vi "Sort Modules.vi"(8 "error in (no error)":errorcluster, 10 "Modules":refnum<class "Module.lvclass">[](array[class]), 11 "Block Diagram in":refnum<class "Block Diagram.lvclass">) -> (0 "error out":errorcluster, 3 "Block Diagram out":refnum<class "Block Diagram.lvclass">)   [LabVIEW 2015, in "Block Diagram.lvclass"]
uses:
  Block Diagram.lvclass
  Module/Module/Module.lvclass
  Block Diagram.lvclass/Block Diagram.ctl
  Structures/Structures.lvclass/Structures.ctl
  Structures/Read Name.vi
  Module Loop/Write Modules.vi
  Module Loop/Module Loop.lvclass
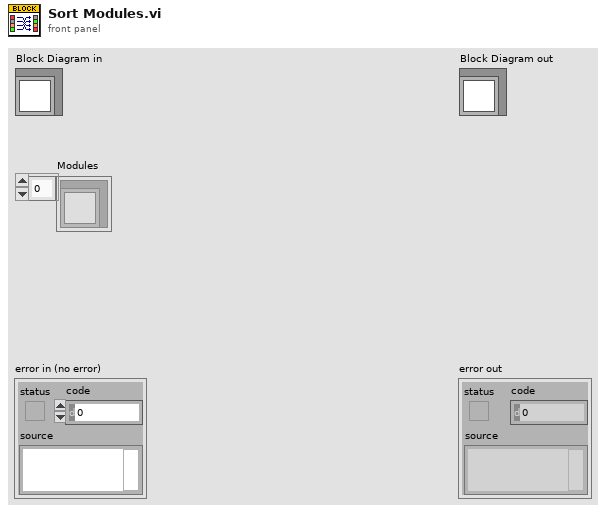
[diagram p1: front panel]
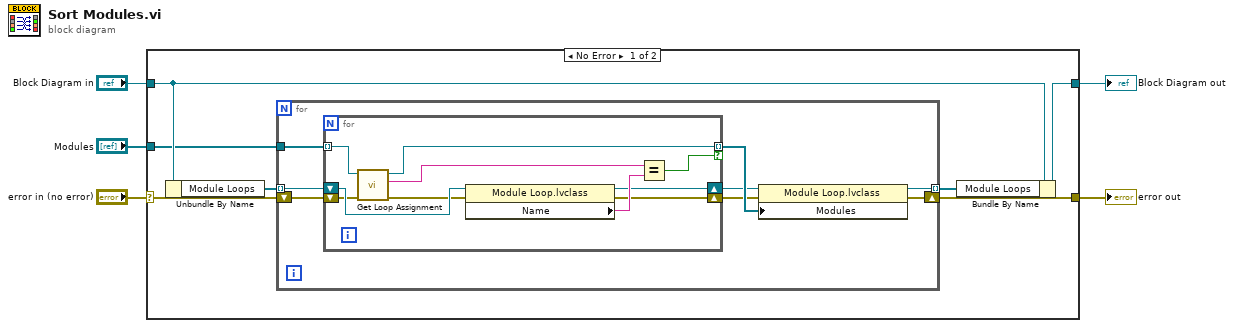
[diagram p0: block diagram]
diagram:
  n1 = case shown="No Error" "error in (no error)" {
    selector: "error in (no error)" -> [w7 w32]
    tunnel: [w6 w32] -> w4
    tunnel: [w12 w31] -> w2
    tunnel: "Block Diagram in" -> [w11 w31]
    tunnel: "Modules" -> [w8 _]
    frame No Error {
      n2 = Unbundle By Name(w11) -> ("Module Loops"=w10:refnum<class "Module Loop.lvclass">[])
      n3 = for {
        tunnel: w8 -> [w20]
        tunnel: w10 -> [w18] mode=indexing
        tunnel: [w17] -> w9 mode=indexing
        shift-right: [w15] -> w6
        shift-left: w7 -> [w14]
        n4 = for {
          tunnel: w20 -> [w25] mode=indexing
          tunnel: [w28] -> w19 mode=indexing if=w27
          shift-right: [w21] -> w16
          shift-left: w14 -> [w26]
          shift-right: [w23] -> w13
          shift-left: w18 -> [w30]
          n5 = call "Get Loop Assignment.vi"("error in (no error)"=w26, "Module in"=w25) -> ("error out"=w22:errorcluster, "Loop Assignment"=w29:string, "Module out"=w28:refnum<class "Module.lvclass">)  [unwired: 7 in]
          n6 = property class="Module Loop.lvclass"(reference=w30, error in=w22) -> (reference out=w23:refnum<class "Module Loop.lvclass">, error out=w21:errorcluster, "Name"=w24:string)
          n7 = Equal?(x=w29, y=w24) -> (x = y?=w27:bool)
        }
        n8 = property class="Module Loop.lvclass"(reference=w13, error in=w16, "Modules"=w19) -> (reference out=w17:refnum<class "Module Loop.lvclass">, error out=w15:errorcluster)
      }
      n9 = Bundle By Name(cluster=w11, "Module Loops"=w9) -> (w12:refnum<class "Block Diagram.lvclass">)
    }
    frame Error {
    }
  }
  "error out" <- w4
  "Block Diagram out" <- w2
